vi "Status Handler.vi"(0 "Variable Index":i32, 1 "Action":T3, 5 "End Tid":dbl, 7 "Value":T1, 9 "Upd freq":T2, 11 "error in (no error)":errorcluster, 12 "Start tid(buff size":dbl) -> (3 "Indexes":i32[](array[numeric]), 6 "Value out":T1, 10 "Values":T1[](array[typedef]), 14 "Numb var":i32, 15 "error out":errorcluster)   [LabVIEW 2011]
uses:
  Action Analog Handler.ctl
  Status Digitalish.ctl
  Update frequensies.ctl
  Status Psudo WF.ctl
panel:
  out "Waveform":waveform(u8)
  in  "Status in":T1
  out "Time Stamp":timestamp
  # "OBS, \nBruk Value som oppdaterings frekvens \nunder reg new var."
  # "Vurder å inkluder en Digital in\nFaktisk pri?"
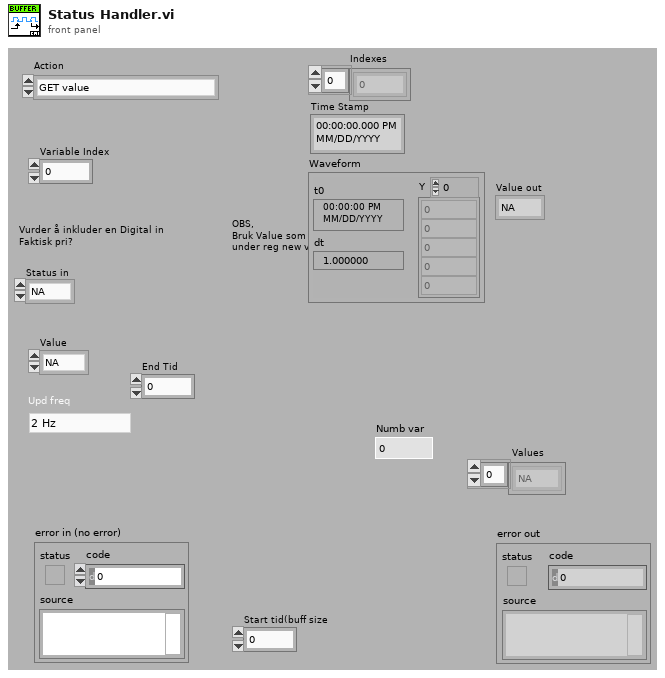
[diagram p1: front panel]
types:
  T1 = typedef "Status Digitalish.ctl" = enum16{"NA", "False", "True"}
  T2 = typedef "Update frequensies.ctl" = enum16{"2 Hz", "1 Hz", "0.1 Hz"}
  T3 = typedef "Action Analog Handler.ctl" = enum16{"GET value", "GET Single Frequenzy", "GET All Values", "GET Waveform", "Get Numb Var", "SET Value", "START Buffer", "REG Variable", "BUF size(total antal sekund)", "PULS", "Get a Value at time", "Set initial waveform"}
  T4 = typedef "Status Psudo WF.ctl" = cluster{"\ndata":T1[], "Index":i32, "Upd freq":T2, "Last index time":dbl, "Rounded":bool}
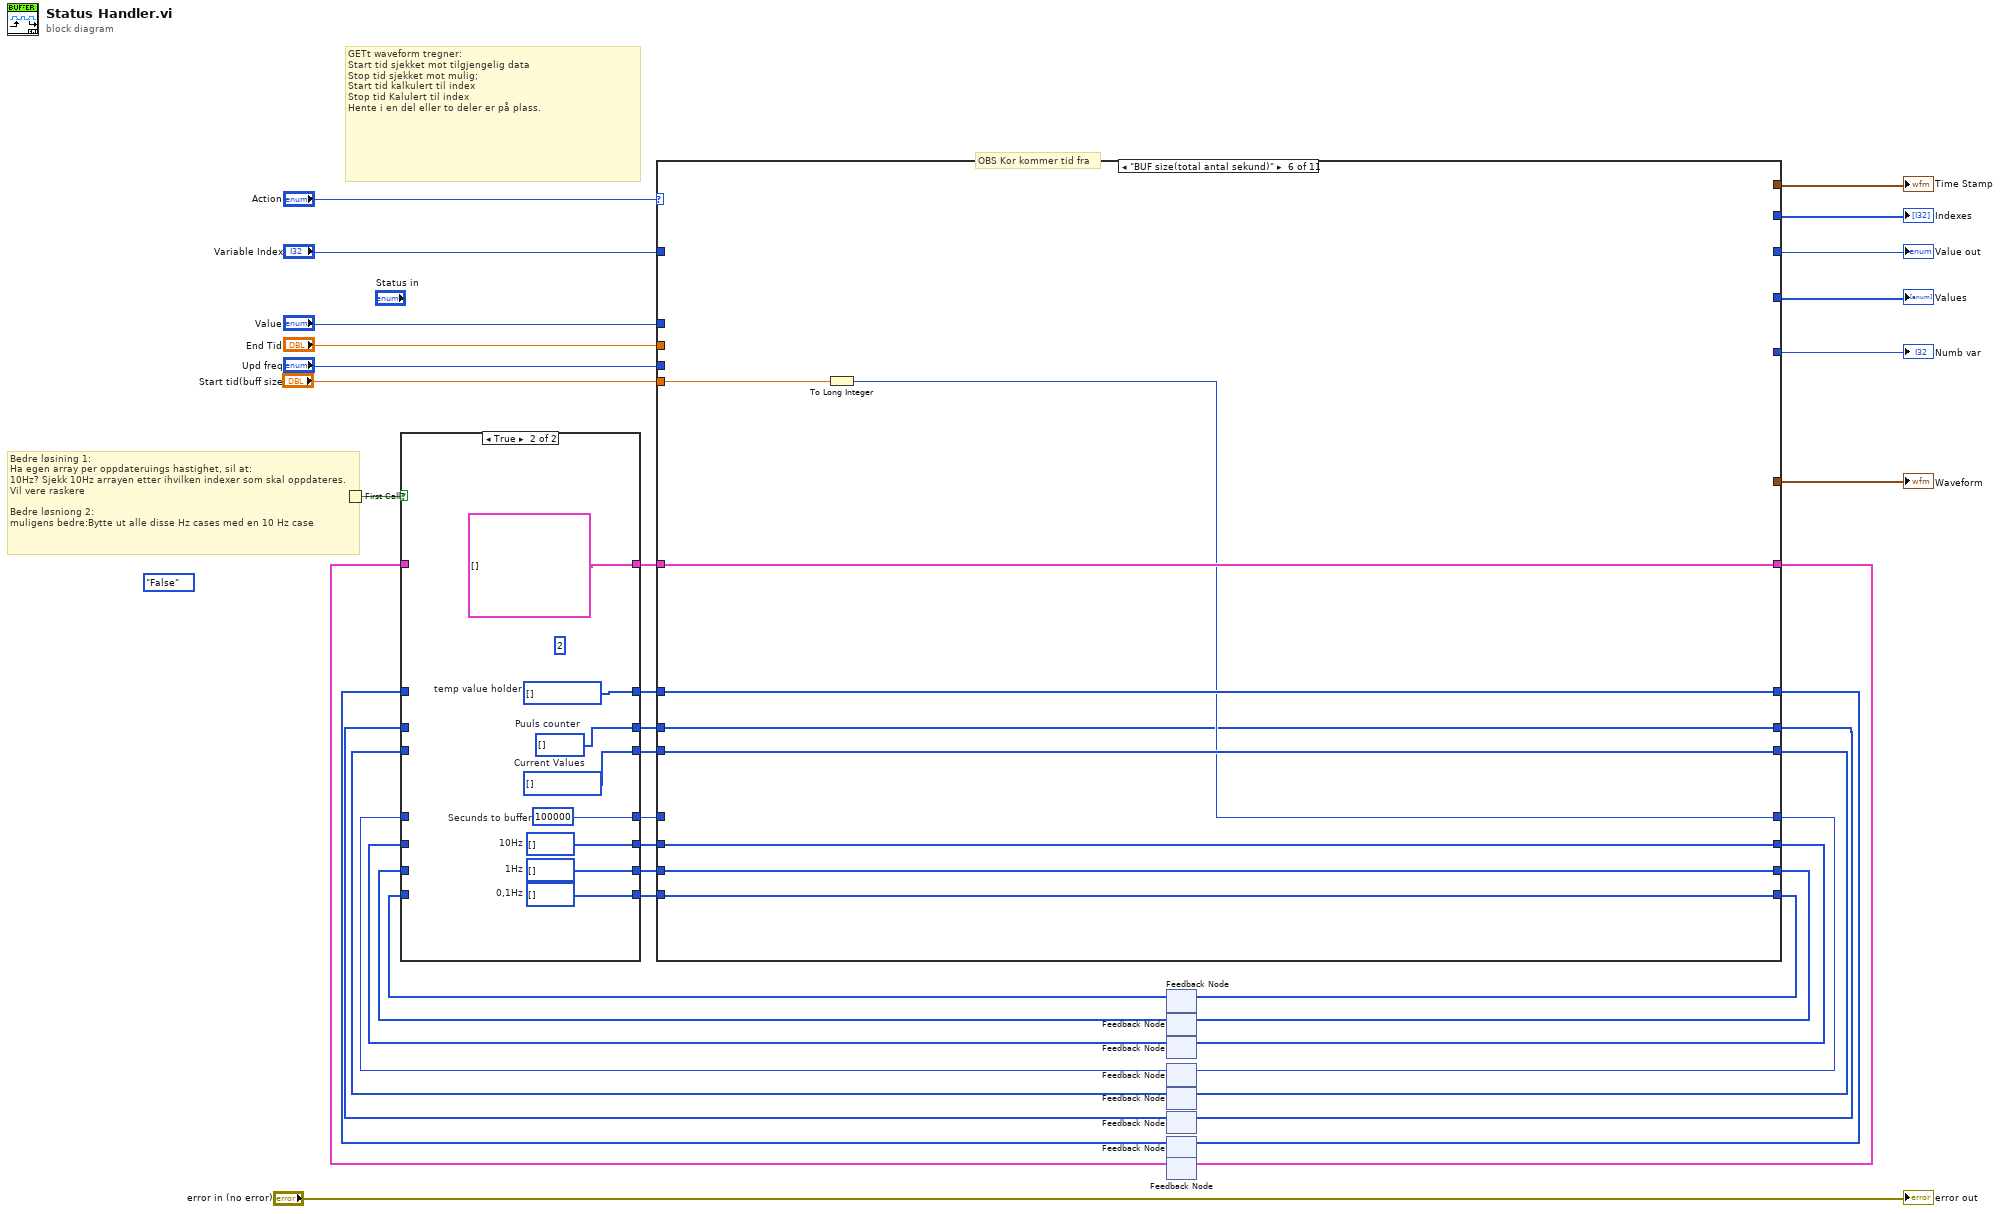
[diagram p0: block diagram]
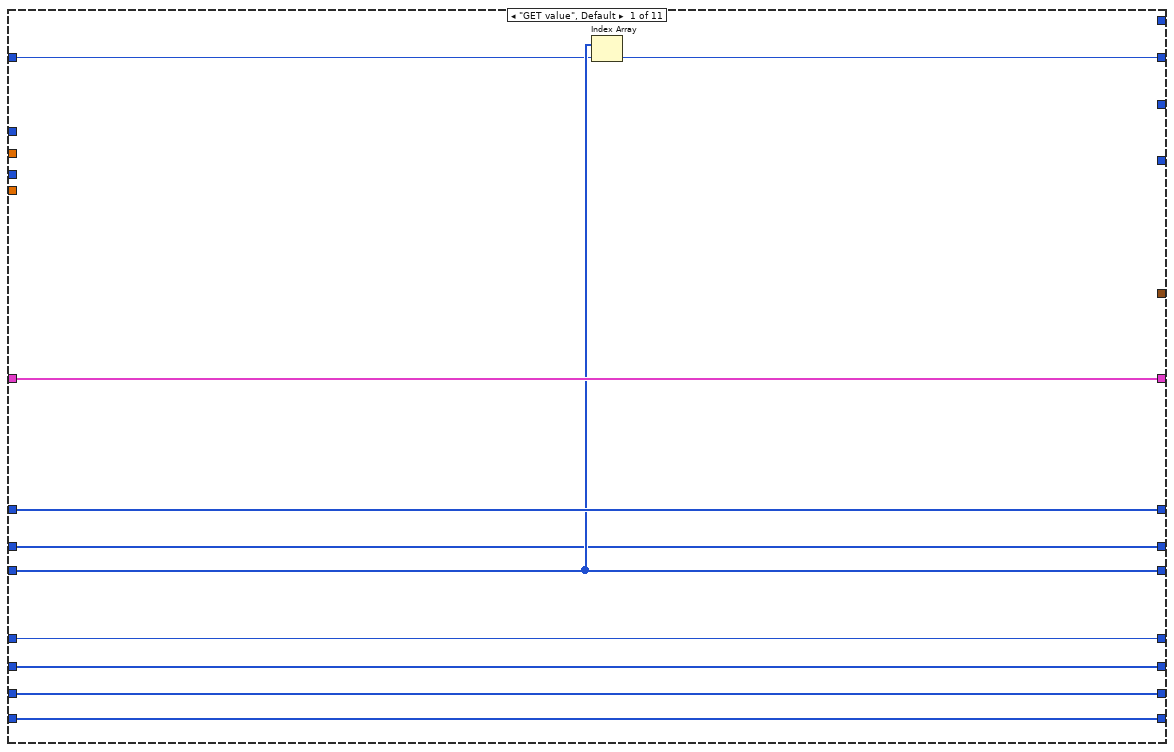
[diagram p3: hidden frame]
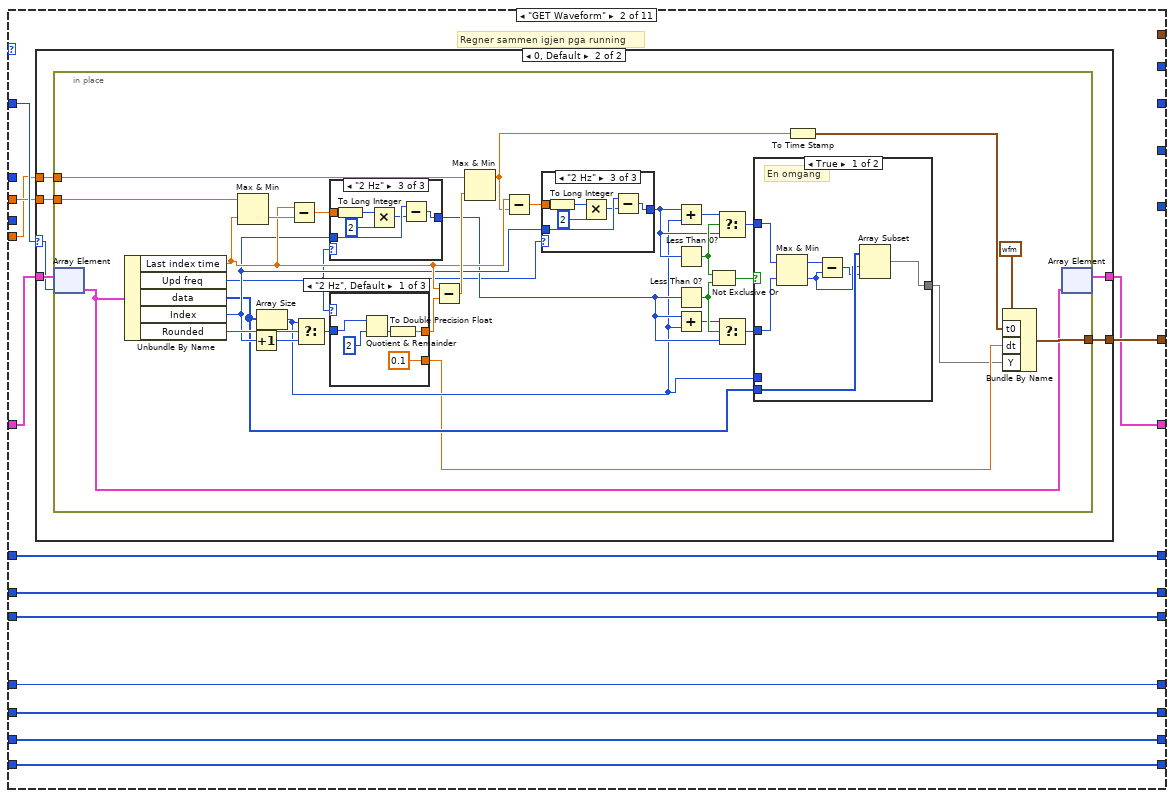
[diagram p4: hidden frame]
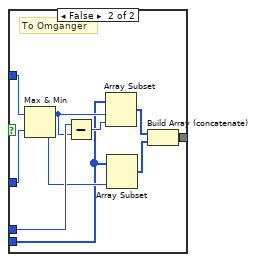
[diagram p6: hidden frame]
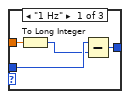
[diagram p7: hidden frame]
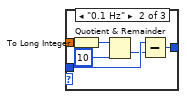
[diagram p8: hidden frame]
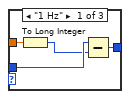
[diagram p9: hidden frame]
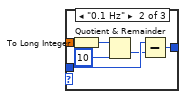
[diagram p10: hidden frame]
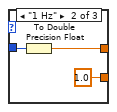
[diagram p11: hidden frame]
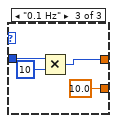
[diagram p12: hidden frame]
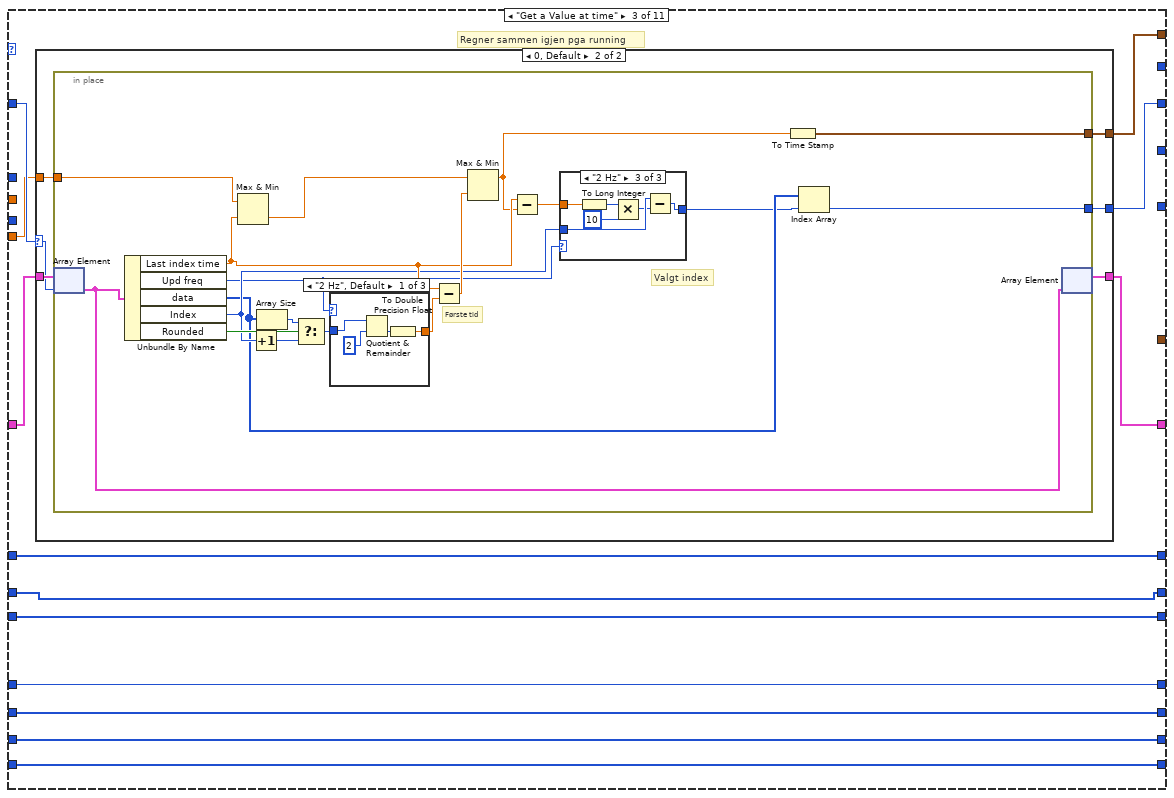
[diagram p13: hidden frame]
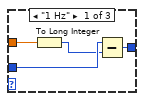
[diagram p15: hidden frame]
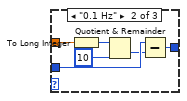
[diagram p16: hidden frame]
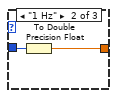
[diagram p17: hidden frame]
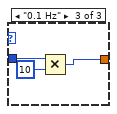
[diagram p18: hidden frame]
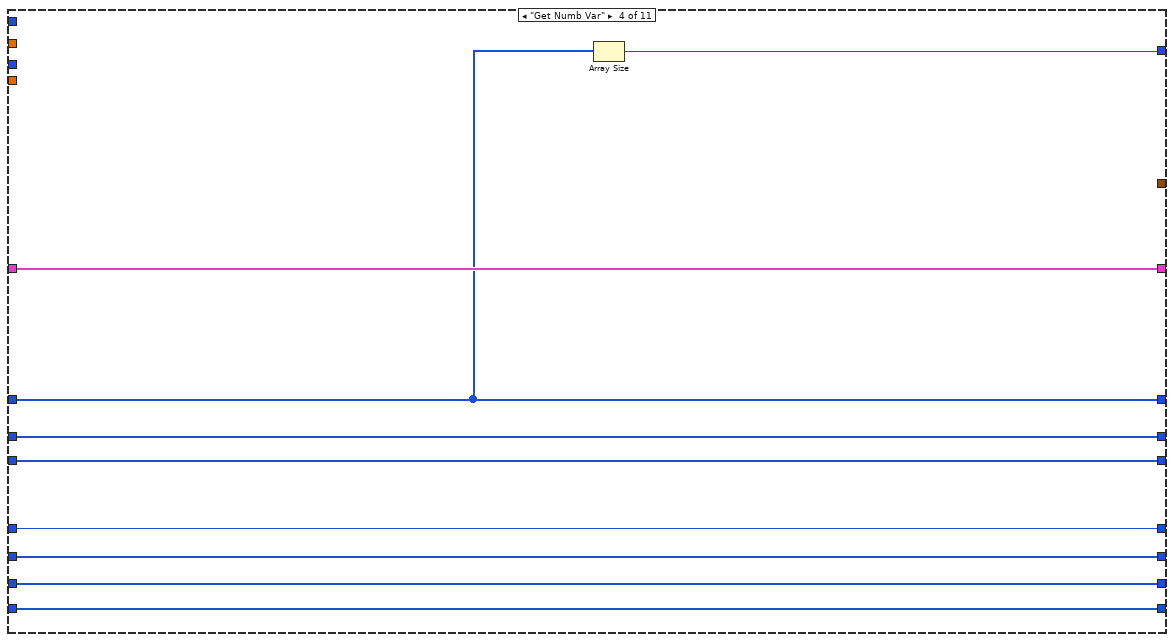
[diagram p19: hidden frame]
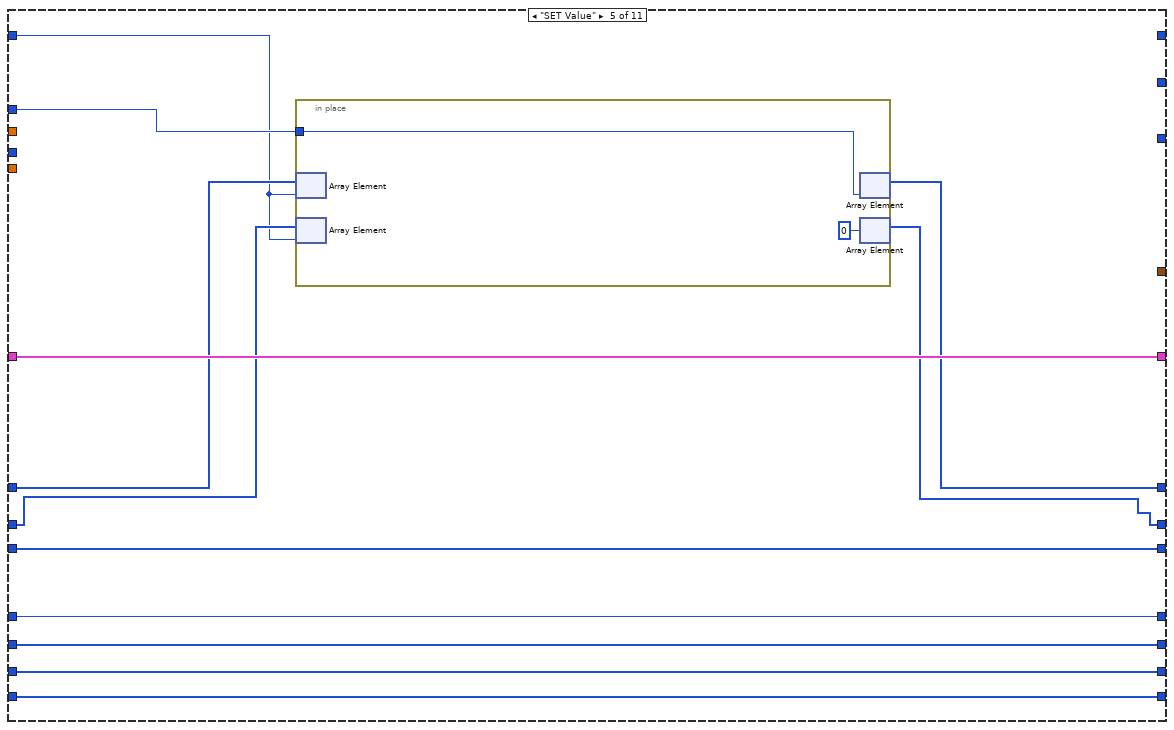
[diagram p20: hidden frame]
diagram:
  (unwired) Status_Digitalish."False" ("Status")
  # "GETt waveform tregner:\nStart tid sjekket mot tilgjengelig data\nStop tid sjekket mot mulig;\nStart tid kalkulert til index\nStop tid Kalulert til index\nHente i en del eller to deler er på plass."
  # "OBS Kor kommer tid fra"
  # "Bedre løsining 1:\nHa egen array per oppdateruings hastighet, sil at:\n10Hz? Sjekk 10Hz arrayen etter ihvilken indexer som skal oppdateres.\nVil vere raskere\n\nBedre løsniong 2:\nmuligens bedre:Bytte ut alle disse Hz cases med en 10 Hz case"
  n1 = First Call?() -> (First Call?: T/F=w35:bool)
  n2 = feedback #1() -> (w12:i32[])  [unwired: 1 in]
  n3 = feedback #2() -> (w13:i32[])  [unwired: 1 in]
  n4 = feedback #3() -> (w14:i32[])  [unwired: 1 in]
  n5 = feedback #4() -> (w11:i32)  [unwired: 1 in]
  n6 = feedback #5() -> (w28:T1[])  [unwired: 1 in]
  n7 = feedback #6() -> (w1:u16[])  [unwired: 1 in]
  n8 = feedback #7() -> (w29:T1[])  [unwired: 1 in]
  n9 = feedback #8() -> (w36:T4[])  [unwired: 1 in]
  n10 = case shown="True" w35 {
    tunnel: w36 -> [w46 _]
    tunnel: [w46 T4[] []] -> w5
    tunnel: [w45 w54] -> w33
    tunnel: [w44 w53] -> w32
    tunnel: w29 -> [w45 _]
    tunnel: w28 -> [w44 _]
    tunnel: [w40 w52] -> w26
    tunnel: [w43 w51] -> w20
    tunnel: [w42 w50] -> w17
    tunnel: [w41 w49] -> w15
    tunnel: w14 -> [w43 _]
    tunnel: w13 -> [w42 _]
    tunnel: w12 -> [w41 _]
    tunnel: w11 -> [w40 _]
    tunnel: [w39 w47] -> w3
    tunnel: w1 -> [w39 _]
    frame False {
    }
    frame True {
      w47 = u8[] []  # Puuls counter
      (unwired) u8 2 ("ValDigital - Status value(0 F, 1 T, 2 NA)")
      w49 = i32[] []  # 0,1Hz
      w50 = i32[] []  # 1Hz
      w51 = i32[] []  # 10Hz
      w52 = 100000  # Secunds to buffer
      w53 = T1[] [] items=["NA", "False", "True"]  # Current Values
      w54 = T1[] [] items=["NA", "False", "True"]  # temp value holder
    }
  }
  n11 = case shown="\"BUF size(total antal sekund)\"" "Action" {
    tunnel: [w64 w69 w182 w248 w260 w271 w288 w347 w374 w405 w475] -> w34
    tunnel: w5 -> [w64 w70 w183 w248 w260 w271 w287 w347 w374 w410 w478]
    tunnel: w33 -> [w63 w77 w189 w241 w257 w270 w285 w348 w376 w387 w477]
    tunnel: w32 -> [w62 w76 w188 w247 w259 w269 w283 w354 w370 w406 w476]
    tunnel: [w63 w77 w189 w241 w256 w270 w286 w348 w376 w404 w474] -> w30
    tunnel: [w62 w76 w188 w247 w259 w269 w284 w355 w370 w403 w473] -> w31
    tunnel: [w59 w67 w181 w246 w258 w265 w282 w353 w375 w385 w479] -> w27
    tunnel: w26 -> [w59 w67 w181 w246 w258 _ w282 w353 w375 w385 w479]
    tunnel: "Variable Index" -> [w60 w71 w184 _ w249 _ _ _ _ w386 w469]
    tunnel: "Value" -> [_ _ _ _ w255 _ _ _ _ _ _]
    tunnel: [w61 _ w179 _ _ _ _ _ _ _ _] -> w23
    tunnel: [_ _ _ _ _ _ w276 w345 w370 _ _] -> w22
    tunnel: [_ _ _ w245 _ _ w277 w346 _ _ _] -> w21
    tunnel: w20 -> [w58 w75 w187 w244 w254 w268 w279 w350 w373 w399 w472]
    tunnel: [w58 w75 w187 w244 w254 w268 w279 w350 w373 w393 w472] -> w19
    tunnel: [w57 w74 w186 w243 w253 w267 w281 w352 w372 w390 w471] -> w18
    tunnel: w17 -> [w57 w74 w186 w243 w253 w267 w281 w352 w372 w398 w471]
    tunnel: [w56 w73 w185 w242 w252 w266 w280 w351 w371 w388 w470] -> w16
    tunnel: w15 -> [w56 w73 w185 w242 w252 w266 w280 w351 w371 w397 w470]
    tunnel: [_ w72 _ _ _ _ _ _ _ _ _] -> w4
    tunnel: "Upd freq" -> [_ _ _ _ _ _ w278 w349 _ w382 _]
    tunnel: [_ _ _ _ _ _ w275 w344 w369 _ _] -> w9
    tunnel: "End Tid" -> [_ w68 _ _ _ _ _ _ _ _ _]
    tunnel: [_ _ w180 _ _ _ _ _ _ _ _] -> w7
    tunnel: "Start tid(buff size" -> [_ w66 w178 _ _ w264 w274 _ _ _ _]
    tunnel: w3 -> [w55 w65 w177 w240 w251 w263 w273 w343 w368 w380 w468]
    tunnel: [w55 w65 w177 w240 w250 w263 w272 w343 w368 w379 w467] -> w2
    frame "GET value", Default {
      n12 = Index Array(array=w62, index=w60) -> (element=w61:T1)
    }
    frame "GET Waveform" {
      # "Regner sammen igjen pga running"
      n13 = case shown="0, Default" w71 {
        selector: w71 -> [_ w81]
        tunnel: w70 -> [w78 w82]
        tunnel: w66 -> [_ w84]
        tunnel: [_ w83] -> w72
        tunnel: [w78 w80] -> w69
        tunnel: w68 -> [_ w79]
        frame ..-1 {
        }
        frame 0, Default {
          n14 = in-place {
            in-place-border: w84 -> [w113]
            in-place-border: [w115] -> w83
            in-place-border: w79 -> [w112]
            n15 = in-place-array #9(w82, w81) -> (w114:T4)
            n16 = Unbundle By Name(w114) -> ("Last index time"=w104:dbl, "Upd freq"=w88:T2, "data"=w92:T1[], "Index"=w102:i32, "Rounded"=w111:bool)
            n17 = Max & Min(x=w112, y=w104) -> (min(x,y)=w106:dbl)  [unwired: 1 out]
            n18 = Increment(x=w102) -> (x+1=w110:i32)
            n19 = Array Size(array=w92) -> (size(s)=w91:i32)
            n20 = Subtract(x=w104, y=w106) -> (x-y=w105:dbl)
            n21 = Select(t=w91, s=w111, f=w110) -> (s? t:f=w109:i32)
            n22 = case shown="\"2 Hz\"" w88 {
              tunnel: w102 -> [w151 w157 w163]
              tunnel: w105 -> [w152 w158 w164]
              tunnel: [w149 w155 w161] -> w99
              frame "1 Hz" {
                n23 = To Long Integer(number=w152) -> (32bit integer=w150:i32)
                n24 = Subtract(x=w151, y=w150) -> (x-y=w149:i32)
              }
              frame "0.1 Hz" {
                n25 = To Long Integer(number=w158) -> (32bit integer=w156:i32)
                n26 = Quotient & Remainder(x=w156, y=10) -> (floor(x/y)=w154:i32)  [unwired: 1 out]
                n27 = Subtract(x=w157, y=w154) -> (x-y=w155:i32)
              }
              frame "2 Hz" {
                n28 = To Long Integer(number=w164) -> (32bit integer=w162:i32)
                n29 = Multiply(x=w162, y=2) -> (x*y=w160:i32)
                n30 = Subtract(x=w163, y=w160) -> (x-y=w161:i32)
              }
            }
            n31 = case shown="\"2 Hz\", Default" w88 {
              tunnel: w109 -> [w169 w172 w176]
              tunnel: [w168 w171 w174] -> w108
              tunnel: [0.1 ("dt") 1.0 ("dt") 10.0 ("dt")] -> w87
              frame "2 Hz", Default {
                n32 = Quotient & Remainder(x=w169, y=2 ("x")) -> (floor(x/y)=w167:i32)  [unwired: 1 out]
                n33 = To Double Precision Float(number=w167) -> (double precision float=w168:dbl)
              }
              frame "1 Hz" {
                n34 = To Double Precision Float(number=w172) -> (double precision float=w171:dbl)
              }
              frame "0.1 Hz" {
                n35 = Multiply(x=w176, y=10) -> (x*y=w174:i32)
              }
            }
            n36 = Subtract(x=w104, y=w108) -> (x-y=w107:dbl)
            n37 = Max & Min(x=w113, y=w107) -> (max(x,y)=w90:dbl)  [unwired: 1 out]
            n38 = Subtract(x=w104, y=w90) -> (x-y=w103:dbl)
            n39 = case shown="\"2 Hz\"" w88 {
              tunnel: w102 -> [w135 w141 w147]
              tunnel: w103 -> [w136 w142 w148]
              tunnel: [w133 w139 w145] -> w96
              frame "1 Hz" {
                n40 = To Long Integer(number=w136) -> (32bit integer=w134:i32)
                n41 = Subtract(x=w135, y=w134) -> (x-y=w133:i32)
              }
              frame "0.1 Hz" {
                n42 = To Long Integer(number=w142) -> (32bit integer=w140:i32)
                n43 = Quotient & Remainder(x=w140, y=10) -> (floor(x/y)=w138:i32)  [unwired: 1 out]
                n44 = Subtract(x=w141, y=w138) -> (x-y=w139:i32)
              }
              frame "2 Hz" {
                n45 = To Long Integer(number=w148) -> (32bit integer=w146:i32)
                n46 = Multiply(x=w146, y=2) -> (x*y=w144:i32)
                n47 = Subtract(x=w147, y=w144) -> (x-y=w145:i32)
              }
            }
            n48 = Add(x=w96, y=w91) -> (x+y=w97:i32)
            n49 = Less Than 0?(x=w96) -> (x < 0?=w101:bool)
            n50 = Less Than 0?(x=w99) -> (x < 0?=w100:bool)
            n51 = Add(x=w99, y=w91) -> (x+y=w98:i32)
            n52 = Not Exclusive Or(1:w100, 2:w101) -> (0:w95:bool)
            n53 = Select(t=w97, s=w101, f=w96) -> (s? t:f=w94:i32)
            n54 = Select(t=w98, s=w100, f=w99) -> (s? t:f=w93:i32)
            n55 = case shown="True" w95 {
              tunnel: w94 -> [w122 w132]
              tunnel: w93 -> [w121 w131]
              tunnel: w92 -> [w119 w126]
              tunnel: [w116 w123] -> w86
              tunnel: w91 -> [_ w130]
              frame True {
                # "En omgang"
                n56 = Max & Min(x=w122, y=w121) -> (max(x,y)=w120:i32, min(x,y)=w118:i32)
                n57 = Subtract(x=w120, y=w118) -> (x-y=w117:i32)
                n58 = Array Subset(array=w119, index=w118, length=w117) -> (w116:T1[])
              }
              frame False {
                # "To Omganger"
                n59 = Max & Min(x=w132, y=w131) -> (max(x,y)=w129:i32, min(x,y)=w127:i32)
                n60 = Subtract(x=w130, y=w129) -> (x-y=w128:i32)
                n61 = Array Subset(array=w126, index=w129, length=w128) -> (w125:T1[])
                n62 = Array Subset(array=w126, length=w127) -> (w124:T1[])  [unwired: 1 in]
                n63 = Build Array (concatenate)(w125, w124) -> (w123:T1[])
              }
            }
            n64 = To Time Stamp(1:w90) -> (0:w89:timestamp)
            n65 = Bundle By Name(cluster=waveform(u8) {"t0"=timestamp(0 s since 1904-01-01), "dt"=1.0, "Y"=[]} ("Waveform"), "t0"=w89, "dt"=w87, "Y"=w86) -> (w115:waveform(u8))
            n66 = in-place-array #9(w114) -> (w80:T4[])  [unwired: 1 out]
          }
        }
      }
    }
    frame "Get a Value at time" {
      # "Regner sammen igjen pga running"
      n67 = case shown="0, Default" w184 {
        selector: w184 -> [_ w194]
        tunnel: w183 -> [w190 w195]
        tunnel: w178 -> [_ w196]
        tunnel: [w190 w193] -> w182
        tunnel: [_ w192] -> w180
        tunnel: [_ w191] -> w179
        frame ..-1 {
        }
        frame 0, Default {
          n68 = in-place {
            in-place-border: w196 -> [w214]
            in-place-border: [w199] -> w192
            in-place-border: [w198] -> w191
            # "Valgt index"
            # "Første tid"
            n69 = in-place-array #10(w195, w194) -> (w197:T4)
            n70 = Unbundle By Name(w197) -> ("Last index time"=w208:dbl, "Upd freq"=w203:T2, "data"=w201:T1[], "Index"=w206:i32, "Rounded"=w213:bool)
            n71 = Max & Min(x=w214, y=w208) -> (min(x,y)=w202:dbl)  [unwired: 1 out]
            n72 = Increment(x=w206) -> (x+1=w212:i32)
            n73 = Array Size(array=w201) -> (size(s)=w205:i32)
            n74 = Select(t=w205, s=w213, f=w212) -> (s? t:f=w211:i32)
            n75 = case shown="\"2 Hz\", Default" w203 {
              tunnel: w211 -> [w234 w236 w239]
              tunnel: [w233 w235 w237] -> w210
              frame "2 Hz", Default {
                n76 = Quotient & Remainder(x=w234, y=2 ("x")) -> (floor(x/y)=w232:i32)  [unwired: 1 out]
                n77 = To Double Precision Float(number=w232) -> (double precision float=w233:dbl)
              }
              frame "1 Hz" {
                n78 = To Double Precision Float(number=w236) -> (double precision float=w235:dbl)
              }
              frame "0.1 Hz" {
                n79 = Multiply(x=w239, y=10) -> (x*y=w237:i32)
              }
            }
            n80 = Subtract(x=w208, y=w210) -> (x-y=w209:dbl)
            n81 = Max & Min(x=w202, y=w209) -> (max(x,y)=w204:dbl)  [unwired: 1 out]
            n82 = Subtract(x=w208, y=w204) -> (x-y=w207:dbl)
            n83 = case shown="\"2 Hz\"" w203 {
              tunnel: w206 -> [w217 w223 w229]
              tunnel: w207 -> [w218 w224 w230]
              tunnel: [w215 w221 w227] -> w200
              frame "1 Hz" {
                n84 = To Long Integer(number=w218) -> (32bit integer=w216:i32)
                n85 = Subtract(x=w217, y=w216) -> (x-y=w215:i32)
              }
              frame "0.1 Hz" {
                n86 = To Long Integer(number=w224) -> (32bit integer=w222:i32)
                n87 = Quotient & Remainder(x=w222, y=10) -> (floor(x/y)=w220:i32)  [unwired: 1 out]
                n88 = Subtract(x=w223, y=w220) -> (x-y=w221:i32)
              }
              frame "2 Hz" {
                n89 = To Long Integer(number=w230) -> (32bit integer=w228:i32)
                n90 = Multiply(x=w228, y=10) -> (x*y=w226:i32)
                n91 = Subtract(x=w229, y=w226) -> (x-y=w227:i32)
              }
            }
            n92 = To Time Stamp(1:w204) -> (0:w199:timestamp)
            n93 = Index Array(array=w201, index=w200) -> (element=w198:T1)
            n94 = in-place-array #10(w197) -> (w193:T4[])  [unwired: 1 out]
          }
        }
      }
    }
    frame "Get Numb Var" {
      n95 = Array Size(array=w241) -> (size(s)=w245:i32)
    }
    frame "SET Value" {
      n96 = in-place {
        in-place-border: w255 -> [w262]
        n97 = in-place-array #11(w257, w249) -> ()  [unwired: 1 out]
        n98 = in-place-array #12(w251, w249) -> ()  [unwired: 1 out]
        n99 = in-place-array #11(w262) -> (w256:T1[])  [unwired: 1 out]
        n100 = in-place-array #12(u8 0 ("element")) -> (w250:u16[])  [unwired: 1 out]
      }
    }
    frame "BUF size(total antal sekund)" {
      n101 = To Long Integer(number=w264) -> (32bit integer=w265:i32)
    }
    frame "PULS" {
      n102 = case shown="\"0.1 Hz\"" w278 {
        tunnel: w279 -> [_ w291 _]
        tunnel: w281 -> [_ _ w292]
        tunnel: w280 -> [w290 _ _]
        tunnel: [w290 w291 w292] -> w275
        frame "0.1 Hz" {
        }
        frame "2 Hz" {
        }
        frame "1 Hz" {
        }
      }
      n103 = Empty Array?(array=w275) -> (empty?=w289:bool)
      n104 = case shown="True" w289 {
        tunnel: [w299 w342] -> w288
        tunnel: w287 -> [w301 w342]
        tunnel: [w298 w341] -> w286
        tunnel: w285 -> [w302 w341]
        tunnel: [w297 w340] -> w284
        tunnel: w283 -> [w303 w340]
        tunnel: w275 -> [w300 _]
        tunnel: w274 -> [w296 _]
        tunnel: [w295 _] -> w276
        tunnel: w273 -> [w294 w339]
        tunnel: [w293 w339] -> w272
        frame False {
          n105 = for {
            tunnel: w300 -> [w305] mode=indexing
            shift-right: [w309] -> w299
            shift-left: w301 -> [w310]
            shift-right: [w311] -> w298
            shift-left: w302 -> [w312]
            shift-right: [w313] -> w297
            shift-left: w303 -> [w314]
            tunnel: w296 -> [w308]
            tunnel: [w307] -> w295 mode=indexing
            shift-right: [w304] -> w293
            shift-left: w294 -> [w306]
            n106 = in-place {
              in-place-border: w308 -> [w323]
              in-place-border: [w316] -> w307
              # "Sets data to NaN if data hasn't been updated\nsince the last 5 pulses"
              n107 = in-place-array #13(w310, w305) -> (w325:T4)
              n108 = in-place-array #14(w312, w305) -> (w316:T1)
              n109 = in-place-array #15(w306, w305) -> (w318:u16)
              n110 = in-place-array #16(w314, w305) -> ()  [unwired: 1 out]
              n111 = in-place {
                in-place-border: w316 -> [w330]
                in-place-border: w323 -> [w329]
                # "Antall skal ikke endre seg"
                n112 = in-place-cluster #17(w325) -> ("data"=w333:T1[], "Index"=w331:i32, "Rounded"=w328:bool)  [unwired: 1 out]
                n113 = in-place {
                  in-place-border: w330 -> [w338]
                  n114 = in-place-array #18(w333, w331) -> ()  [unwired: 1 out]
                  n115 = in-place-array #18(w338) -> (w332:T1[])  [unwired: 1 out]
                }
                n116 = Array Size(array=w333) -> (size(s)=w337:i32)
                n117 = Increment(x=w331) -> (x+1=w336:i32)
                n118 = Greater Or Equal?(x=w336, y=w337) -> (x >= y?=w327:bool)
                n119 = Select(t=0, s=w327, f=w336) -> (s? t:f=w334:i32)
                n120 = Or(x=w327, y=w328) -> (x .or. y?=w326:bool)
                n121 = in-place-cluster #17("Last index time"=w329, "data"=w332, "Index"=w334, "Rounded"=w326) -> (w324:T4)
              }
              n122 = Greater Or Equal?(x=w318, y=u8 5) -> (x >= y?=w321:bool)
              n123 = Select(t=Status_Digitalish."NA", s=w321, f=w316) -> (s? t:f=w315:T1)
              n124 = Increment(x=w318) -> (x+1=w320:u16)
              n125 = Select(t=w318, s=w321, f=w320) -> (s? t:f=w317:u16)
              n126 = in-place-array #13(w324) -> (w309:T4[])  [unwired: 1 out]
              n127 = in-place-array #14(w315) -> (w311:T1[])  [unwired: 1 out]
              n128 = in-place-array #15(w317) -> (w304:u16[])  [unwired: 1 out]
              n129 = in-place-array #16(w316) -> (w313:T1[])  [unwired: 1 out]
            }
          }
        }
        frame True {
          # "Ingen 10 Hzere"
        }
      }
      n130 = Array Size(array=w276) -> (size(s)=w277:i32)
    }
    frame "GET Single Frequenzy" {
      n131 = case shown="\"0.1 Hz\"" w349 {
        tunnel: w350 -> [_ w358 _]
        tunnel: w352 -> [_ _ w359]
        tunnel: w351 -> [w357 _ _]
        tunnel: [w357 w358 w359] -> w344
        frame "0.1 Hz" {
        }
        frame "2 Hz" {
        }
        frame "1 Hz" {
        }
      }
      n132 = Empty Array?(array=w344) -> (empty?=w356:bool)
      n133 = case shown="False" w356 {
        tunnel: [w362 w367] -> w355
        tunnel: w354 -> [w363 w367]
        tunnel: w344 -> [w361 _]
        tunnel: [w360 _] -> w345
        frame False {
          n134 = for {
            shift-right: [w365] -> w362
            shift-left: w363 -> [w365]
            tunnel: w361 -> [w366] mode=indexing
            tunnel: [w364] -> w360 mode=indexing
            n135 = Index Array(array=w365, index=w366) -> (element=w364:T1)
          }
        }
        frame True {
        }
      }
      n136 = Array Size(array=w345) -> (size(s)=w346:i32)
    }
    frame "GET All Values" {
      n137 = for {
        tunnel: w370 -> [_] mode=indexing
        tunnel: [w377] -> w369 mode=indexing
        i -> [w377]
      }
    }
    frame "REG Variable" {
      # "Fjerner den nye, om den ligger i en av listene"
      n138 = To Long Integer(number=w386) -> (32bit integer=w378:i32)
      n139 = Increment(x=w378) -> (x+1=w401:i32)
      n140 = Search 1D Array(1D array=w397, element=w378) -> (index of element=w396:i32)  [unwired: 1 in]
      n141 = Array Size(array=w387) -> (size(s)=w402:i32)
      n142 = Subtract(x=w401, y=w402) -> (x-y=w400:i32)
      n143 = Delete From Array(array=w397, index=w396) -> (array with subset deleted=w389:i32[])  [unwired: 1 in, 1 out]
      n144 = Search 1D Array(1D array=w398, element=w378) -> (index of element=w394:i32)  [unwired: 1 in]
      n145 = case shown="\"1 Hz\"" w382 {
        selector: w382 -> [w411 w415 w419]
        tunnel: w385 -> [w414 w418 w420]
        tunnel: [w412 w416 w420] -> w384
        tunnel: [w411 w415 w419] -> w383
        frame "2 Hz" {
          n146 = Multiply(x=w414, y=2) -> (x*y=w412:i32)
        }
        frame "0.1 Hz" {
          n147 = Quotient & Remainder(x=w418, y=10) -> (floor(x/y)=w416:i32)  [unwired: 1 out]
        }
        frame "1 Hz" {
        }
      }
      n148 = Delete From Array(array=w398, index=w394) -> (array with subset deleted=w391:i32[])  [unwired: 1 in, 1 out]
      n149 = case shown="0" w400 {
        selector: w400 -> [_ w440]
        tunnel: w410 -> [w439 w459]
        tunnel: [w439 w458] -> w409
        tunnel: [w438 w446] -> w408
        tunnel: w387 -> [w438 w456]
        tunnel: [w437 w457] -> w407
        tunnel: w406 -> [w437 w455]
        tunnel: w384 -> [_ w449]
        tunnel: w383 -> [_ w448]
        tunnel: [w436 w445] -> w381
        tunnel: w380 -> [w436 w444]
        frame 0 {
        }
        frame 1, Default {
          w443 = Status_Digitalish."NA"
          n150 = Initialize Array(w443, w449) -> (w451:T1[])
          n151 = Bundle By Name(cluster=T4 {"\ndata"=[], "Index"=0, "Upd freq"=enum."2 Hz", "Last index time"=0.0, "Rounded"=FALSE} ("Cluster"), "data"=w451, "Upd freq"=w448) -> (w450:T4)
          n152 = Initialize Array(w450, w440) -> (w454:T4[])
          n153 = Initialize Array(w443, w440) -> (w453:T1[])
          n154 = Initialize Array(u16 0, w440) -> (w441:u16[])
          n155 = Initialize Array(w443, w440) -> (w452:T1[])
          n156 = Build Array (concatenate)(w459, w454) -> (w458:T4[])
          n157 = Build Array (concatenate)(w456, w453) -> (w446:T1[])
          n158 = Build Array (concatenate)(w444, w441) -> (w445:u16[])
          n159 = Build Array (concatenate)(w455, w452) -> (w457:T1[])
        }
      }
      n160 = Search 1D Array(1D array=w399, element=w378) -> (index of element=w395:i32)  [unwired: 1 in]
      n161 = Delete From Array(array=w399, index=w395) -> (array with subset deleted=w392:i32[])  [unwired: 1 in, 1 out]
      n162 = case shown="\"2 Hz\"" w382 {
        tunnel: [w425 w427 w435] -> w393
        tunnel: w392 -> [w425 w430 w435]
        tunnel: w391 -> [w424 w429 w434]
        tunnel: [w424 w429 w432] -> w390
        tunnel: w389 -> [w423 w428 w433]
        tunnel: [w422 w428 w433] -> w388
        tunnel: w378 -> [w421 w426 w431]
        frame "0.1 Hz" {
          n163 = Build Array (concatenate)(w423, w421) -> (w422:i32[])
        }
        frame "2 Hz" {
          n164 = Build Array (concatenate)(w430, w426) -> (w427:i32[])
        }
        frame "1 Hz" {
          n165 = Build Array (concatenate)(w434, w431) -> (w432:i32[])
        }
      }
      n166 = in-place {
        in-place-border: w384 -> [w464]
        in-place-border: w383 -> [w463]
        w461 = Status_Digitalish."NA"
        (unwired) nan ("element")
        n167 = in-place-array #19(w409, w378) -> ()  [unwired: 1 out]
        n168 = in-place-array #20(w408, w378) -> ()  [unwired: 1 out]
        n169 = in-place-array #21(w381, w378) -> ()  [unwired: 1 out]
        n170 = in-place-array #22(w407, w378) -> ()  [unwired: 1 out]
        n171 = Initialize Array(w461, w464) -> (w466:T1[])
        n172 = Bundle By Name(cluster=T4 {"\ndata"=[], "Index"=0, "Upd freq"=enum."2 Hz", "Last index time"=0.0, "Rounded"=FALSE} ("Cluster"), "data"=w466, "Upd freq"=w463) -> (w465:T4)
        n173 = in-place-array #19(w465) -> (w405:T4[])  [unwired: 1 out]
        n174 = in-place-array #20(w461) -> (w404:T1[])  [unwired: 1 out]
        n175 = in-place-array #21(u16 0) -> (w379:u16[])  [unwired: 1 out]
        n176 = in-place-array #22(w461) -> (w403:T1[])  [unwired: 1 out]
      }
    }
    frame "START Buffer" {
      n177 = in-place {
        w481 = Status_Digitalish."NA"
        (unwired) FALSE
        n178 = in-place-array #23(w478, w469) -> (w486:T4)
        n179 = in-place-array #24(w477, w469) -> ()  [unwired: 1 out]
        n180 = in-place-array #25(w468, w469) -> ()  [unwired: 1 out]
        n181 = in-place-array #26(w476, w469) -> ()  [unwired: 1 out]
        n182 = Unbundle By Name(w486) -> ("data"=w485:T1[], "Upd freq"=w480:T2)
        n183 = Array Size(array=w485) -> (size(s)=w484:i32)
        n184 = Initialize Array(w481, w484) -> (w487:T1[])
        n185 = Bundle By Name(cluster=T4 {"\ndata"=[], "Index"=0, "Upd freq"=enum."2 Hz", "Last index time"=0.0, "Rounded"=FALSE} ("Cluster"), "data"=w487, "Upd freq"=w480) -> (w483:T4)
        n186 = in-place-array #23(w483) -> (w475:T4[])  [unwired: 1 out]
        n187 = in-place-array #24(w481) -> (w474:T1[])  [unwired: 1 out]
        n188 = in-place-array #25(w481) -> (w467:u16[])  [unwired: 1 out]
        n189 = in-place-array #26(w481) -> (w473:T1[])  [unwired: 1 out]
      }
    }
  }
  "Values" <- w22
  "Value out" <- w23
  "Numb var" <- w21
  "Indexes" <- w9
  "Time Stamp" <- w7
  "Waveform" <- w4
  n190 = feedback-in #1(w16) -> ()
  n191 = feedback-in #2(w18) -> ()
  n192 = feedback-in #3(w19) -> ()
  n193 = feedback-in #4(w27) -> ()
  n194 = feedback-in #5(w31) -> ()
  n195 = feedback-in #6(w2) -> ()
  n196 = feedback-in #7(w30) -> ()
  n197 = feedback-in #8(w34) -> ()
  "error out" <- "error in (no error)"
